vi "Append or Replace Array Element Example 01.vi"() -> ()   [LabVIEW 2009]
uses:
  Append or Replace Array Element/Append or Replace 2D Array Element (Boolean).vi
panel:
  out "Array with Element (1,1) Changed":bool[][](array[boolean])
  in  "Array":bool[][](array[boolean])=[[TRUE, FALSE, FALSE, FALSE, TRUE, FALSE], [FALSE, FALSE, TRUE, FALSE, FALSE, FALSE], [TRUE, FALSE, FALSE, FALSE, TRUE, TRUE], [FALSE, TRUE, FALSE, TRUE, FALSE, FALSE]]
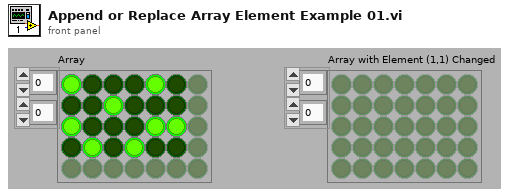
[diagram p1: front panel]
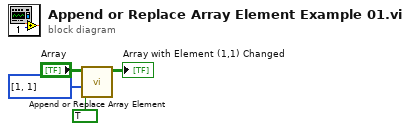
[diagram p0: block diagram]
diagram:
  n1 = call-poly "Append or Replace Array Element.vi"("Element"=TRUE, "Indices (>=1D)"=i32[] [1, 1], "Array In"="Array") -> ("Array Out"=→"Array with Element (1,1) Changed":bool[][])  [unwired: 8 in]
